vi "Clamp Set.vi"() -> (3 "End":bool)   [LabVIEW 2013]
doc: "This VI is used in 2-ball Autonomous Mode in order to get the second ball from behind the robot."
uses:
  <vilib>/Rock Robotics/WPI/Solenoid/Deprecated/WPI_SolenoidSetBool.vi
panel:
  out "State":T1(ring)
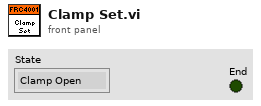
[diagram p1: front panel]
types:
  T1 = enum16{"Clamp Open", "Clamp Down", "Clamp Close", "Clamp Raise"}
  T2 = enum16{"Clamp Open", "Clamp Down", "Clamp Close", "Clamp Raise", "Motor Stop"}
  T3 = typedef "WPI_DigitalInputDevRef.ctl" = cluster{"DevStatus":errorcluster, "DIO Channel":T4, "Digital Module":T5}
  T4 = typedef "FPGA_DIOChannel.ctl" = enum8{"DIO 1", "DIO 2", "DIO 3", "DIO 4", "DIO 5", "DIO 6", "DIO 7", "DIO 8", "DIO 9", "DIO 10", "DIO 11", "DIO 12", "DIO 13", "DIO 14", "Invalid"}
  T5 = typedef "FPGA_TypedefDigitalModule.ctl" = enum16{"Digital Module 1", "Digital Module 2"}
  T6 = typedef "WPI_SolenoidDevRef.ctl" = cluster{"DevStatus":errorcluster, "Solenoid Module":T7, "Forward Solenoid Channel":T8, "Reverse Solenoid Channel":T8}
  T7 = typedef "FPGA_TypedefSolenoidModule.ctl" = enum16{"Solenoid Module 1", "Solenoid Module 2"}
  T8 = typedef "WPI_SolenoidChannel.ctl" = enum8{"Solenoid 1", "Solenoid 2", "Solenoid 3", "Solenoid 4", "Solenoid 5", "Solenoid 6", "Solenoid 7", "Solenoid 8", "Invalid"}
  T9 = typedef "WPI_MotorControlDeviceRef.ctl" = cluster{"DeviceStatus":errorcluster, "Type":enum16{"PWM", "CAN"}, "PWM":cluster{"Digital Module":T5, "PWM Channel":T10, "DeadBand":T11}, "CAN":cluster{"Device Number":u8, "Control Mode":T12, "Semaphore":T13, "Max Vout":dbl}, "Invert":bool, "TransformRef":T14, "InvTransformRef":T14}
  T10 = typedef "FPGA_DIOPWMChannel.ctl" = enum8{"PWM 1", "PWM 2", "PWM 3", "PWM 4", "PWM 5", "PWM 6", "PWM 7", "PWM 8", "PWM 9", "PWM 10", "Invalid"}
  T11 = typedef "WPI_PWMDeadband.ctl" = cluster{"Name":string, "maxPositivePwm":i32, "minPositivePwm":i32, "centerPwm":i32, "maxNegativePwm":i32, "minNegativePwm":i32, "angularRange":u16}
  T12 = typedef "WPI_CANJaguar_ControlMode.ctl" = enum8{"Percent VBus", "Current", "Speed", "Position", "Voltage"}
  T13 = typedef "Semaphore RefNum" = refnum<k1>
  T14 = typedef "WPI_PWMTransform_ConPane.ctl" = refnum<vi>
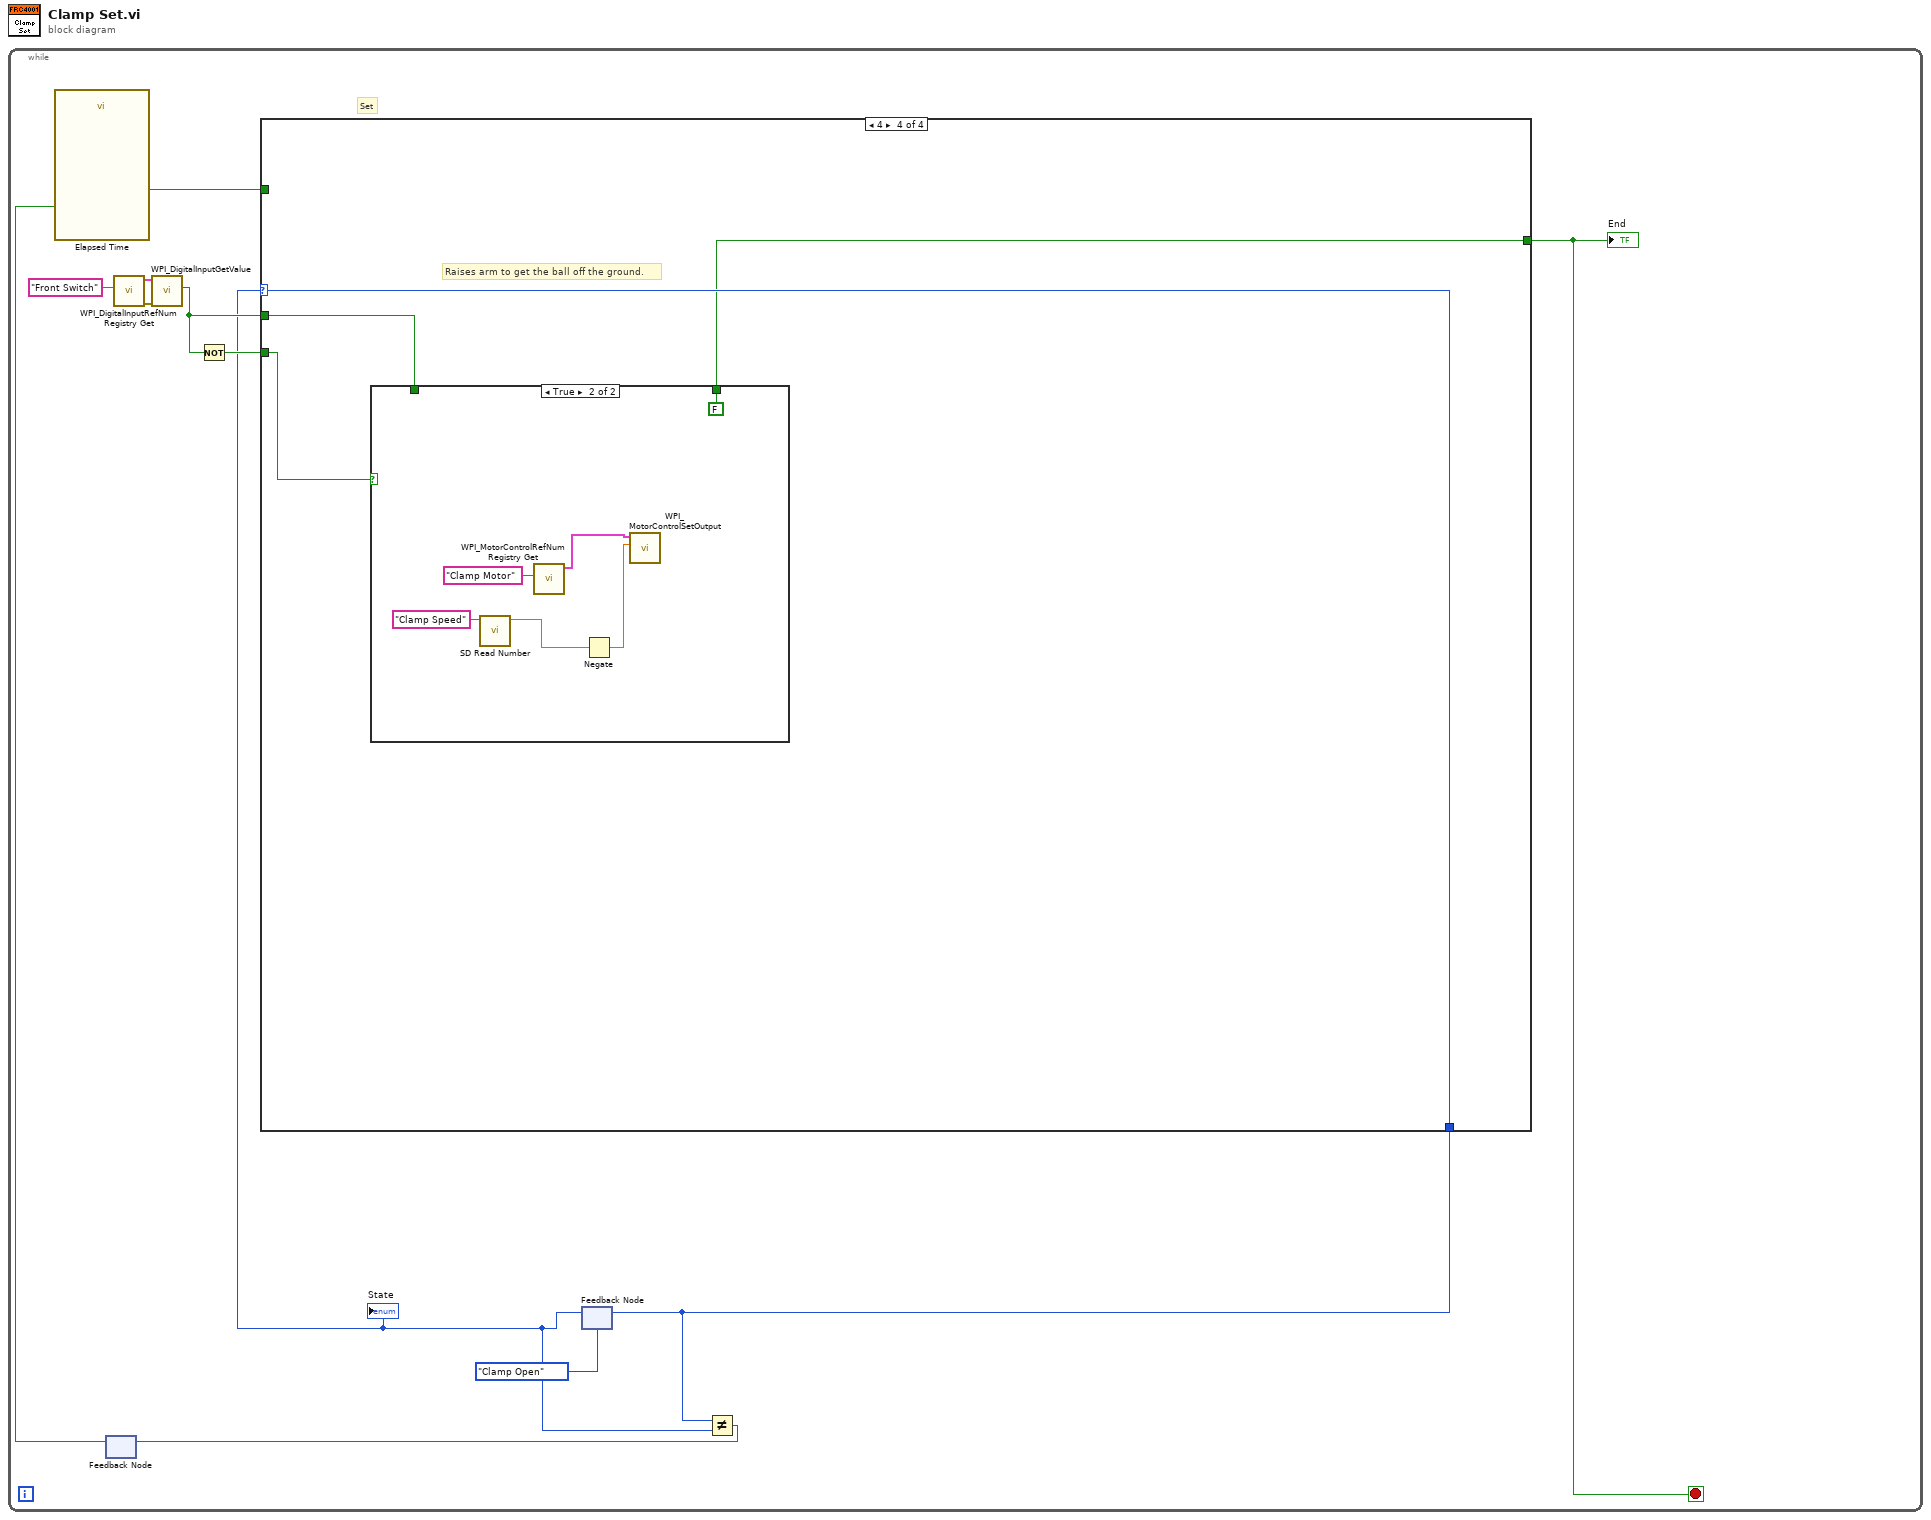
[diagram p0: block diagram]
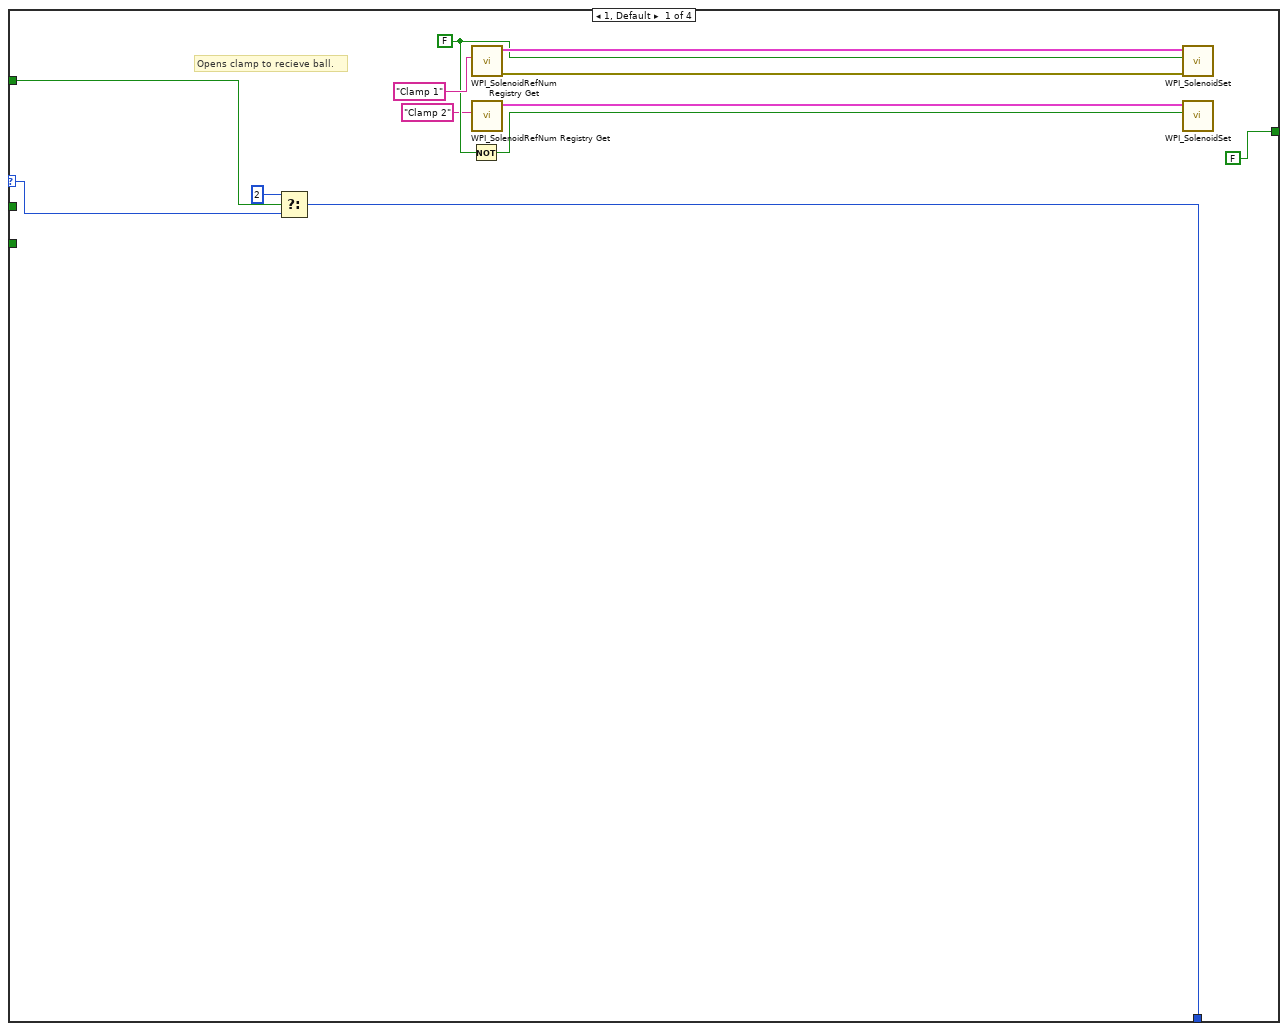
[diagram p2: hidden frame]
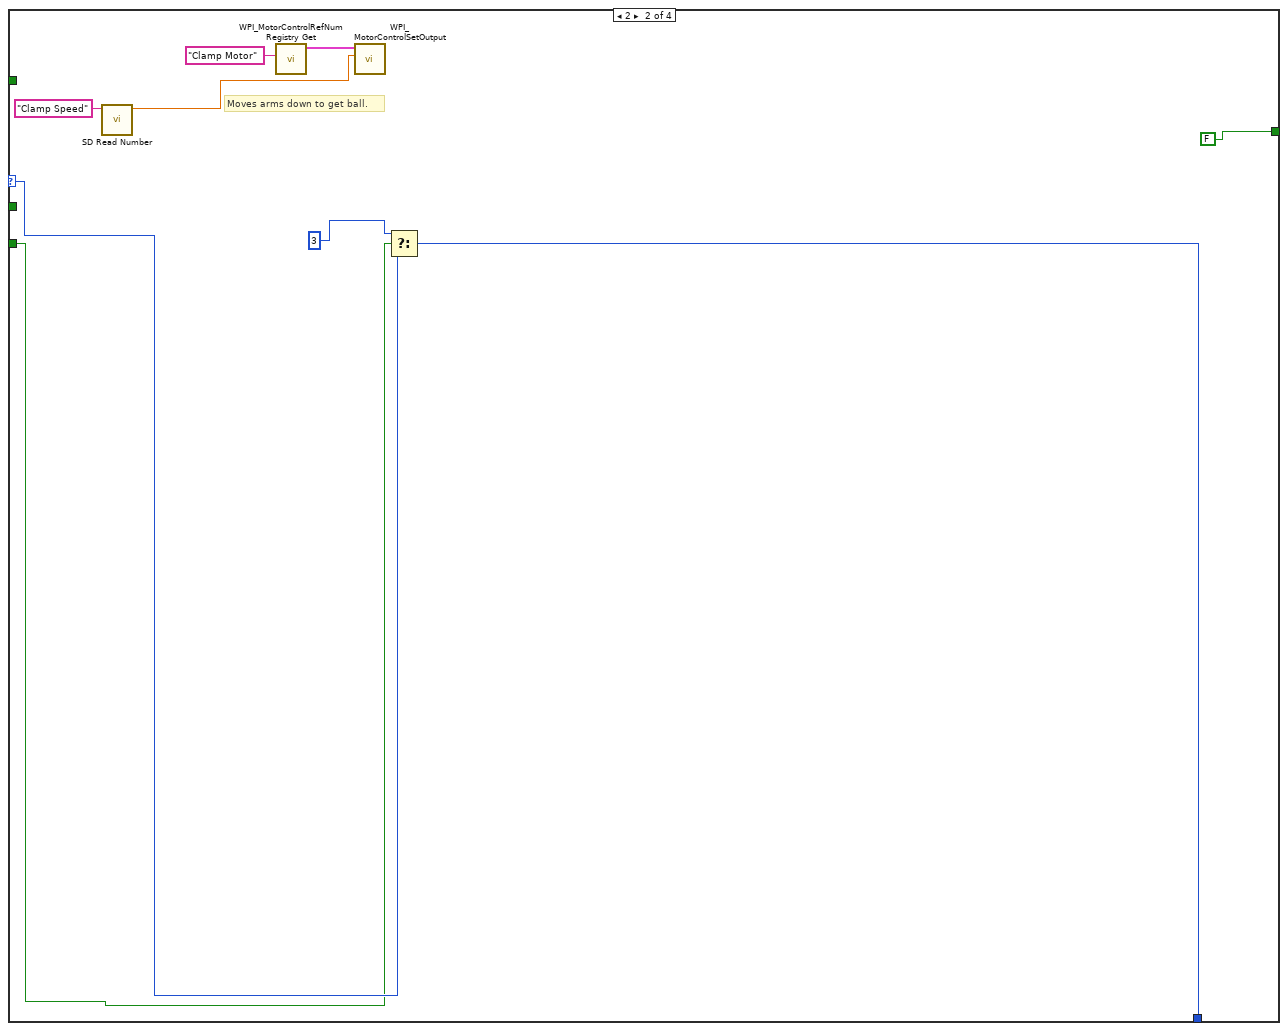
[diagram p3: hidden frame]
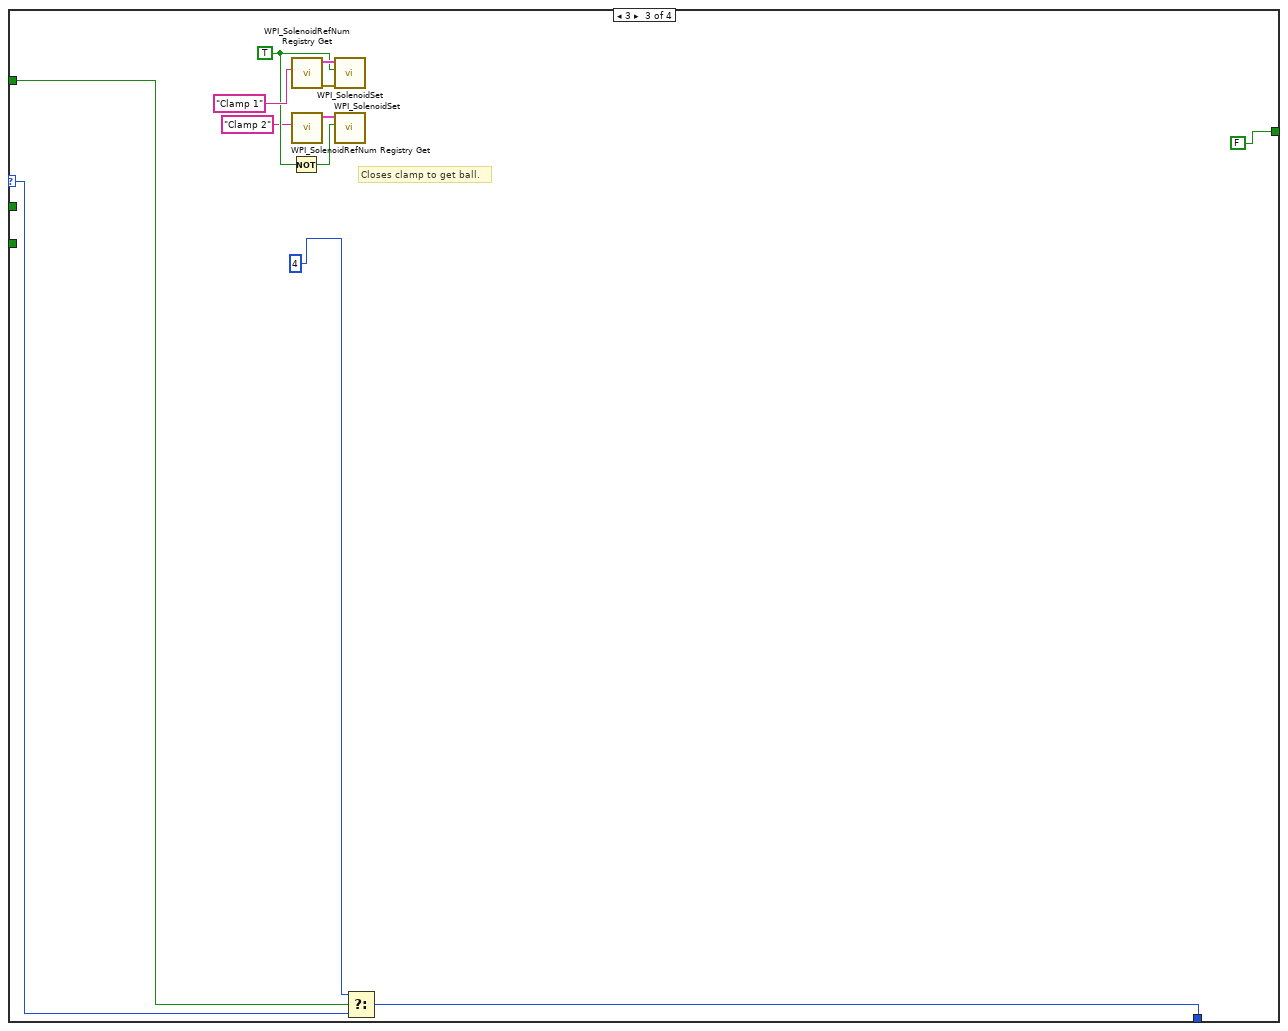
[diagram p4: hidden frame]
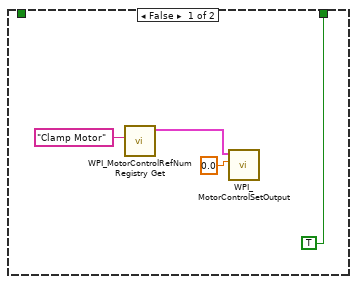
[diagram p5: hidden frame]
diagram:
  n1 = while {
    stop <- w4 stop-if-true
    # "Set"
    n2 = feedback #1() -> (w6:bool)  [unwired: 1 in]
    n3 = call "Elapsed Time"("Reset"=w6) -> ("Time has Elapsed"=w9:bool)  [unwired: 11 in, 7 out]
    n4 = call <vilib>:"WPI_DigitalInputRefNum Registry Get.vi"("refnum name"="Front Switch") -> ("error out"=w11:errorcluster, "DigitalInputDevRef"=w10:T3)  [unwired: 9 in]
    n5 = call <vilib>:"WPI_DigitalInputGetValue.vi"("error in (no error)"=w11, "DigitalInputDevRef"=w10) -> ("Value"=w3:bool)  [unwired: 7 in, 2 out]
    n6 = Not(x=w3) -> (.not. x?=w5:bool)
    n7 = feedback #2(T2."Clamp Open") -> (w1:u16)
    "State" <- w1
    n8 = case shown="4" w1 {
      selector: w1 -> [w23 w32 w44 w49]
      tunnel: [FALSE FALSE FALSE w46] -> w4
      tunnel: [w22 w31 w43 w49] -> w8
      tunnel: w5 -> [_ w28 _ w48]
      tunnel: w9 -> [w14 _ w35 _]
      tunnel: w3 -> [_ _ _ w47]
      frame 1, Default {
        w18 = FALSE
        # "Opens clamp to recieve ball."
        n9 = Select(t=u16 2, s=w14, f=w23) -> (s? t:f=w22:u16)
        n10 = Not(x=w18) -> (.not. x?=w16:bool)
        n11 = call <vilib>:"WPI_SolenoidRefNum Registry Get.vi"("refnum name"="Clamp 1") -> ("error out"=w19:errorcluster, "SolenoidDevRef"=w20:T6)  [unwired: 9 in]
        n12 = call <vilib>:"WPI_SolenoidRefNum Registry Get.vi"("refnum name"="Clamp 2") -> ("SolenoidDevRef"=w17:T6)  [unwired: 9 in, 1 out]
        n13 = call-poly <vilib>:"WPI_SolenoidSet.vi"("error in (no error)"=w19, "Value"=w18, "SolenoidDevRef"=w20) -> ()  [unwired: 7 in, 2 out]
        n14 = call-poly <vilib>:"WPI_SolenoidSet.vi"("Value"=w16, "SolenoidDevRef"=w17) -> ()  [unwired: 8 in, 2 out]
      }
      frame 2 {
        # "Moves arms down to get ball."
        n15 = call <vilib>:"SD Read Number.vi"("Name"="Clamp Speed") -> ("Numeric"=w25:dbl)  [unwired: 8 in, 2 out]
        n16 = call <vilib>:"WPI_MotorControlRefNum Registry Get.vi"("refnum name"="Clamp Motor") -> ("MotorControlDevRef"=w29:T9)  [unwired: 9 in, 1 out]
        n17 = call <vilib>:"WPI_MotorControlSetOutput.vi"("Output"=w25, "MotorControlDevRef"=w29) -> ()  [unwired: 7 in, 3 out]
        n18 = Select(t=u16 3, s=w28, f=w32) -> (s? t:f=w31:u16)
      }
      frame 3 {
        w39 = TRUE
        # "Closes clamp to get ball."
        n19 = Not(x=w39) -> (.not. x?=w37:bool)
        n20 = call <vilib>:"WPI_SolenoidRefNum Registry Get.vi"("refnum name"="Clamp 1") -> ("error out"=w40:errorcluster, "SolenoidDevRef"=w41:T6)  [unwired: 9 in]
        n21 = call <vilib>:"WPI_SolenoidRefNum Registry Get.vi"("refnum name"="Clamp 2") -> ("SolenoidDevRef"=w38:T6)  [unwired: 9 in, 1 out]
        n22 = call-poly <vilib>:"WPI_SolenoidSet.vi"("error in (no error)"=w40, "Value"=w39, "SolenoidDevRef"=w41) -> ()  [unwired: 7 in, 2 out]
        n23 = call-poly <vilib>:"WPI_SolenoidSet.vi"("Value"=w37, "SolenoidDevRef"=w38) -> ()  [unwired: 8 in, 2 out]
        n24 = Select(t=u16 4, s=w35, f=w44) -> (s? t:f=w43:u16)
      }
      frame 4 {
        # "Raises arm to get the ball off the ground."
        n25 = case shown="True" w48 {
          tunnel: w47 -> [_ _]
          tunnel: [TRUE FALSE] -> w46
          frame False {
            n26 = call <vilib>:"WPI_MotorControlRefNum Registry Get.vi"("refnum name"="Clamp Motor") -> ("MotorControlDevRef"=w51:T9)  [unwired: 9 in, 1 out]
            n27 = call <vilib>:"WPI_MotorControlSetOutput.vi"("Output"=0.0, "MotorControlDevRef"=w51) -> ()  [unwired: 7 in, 3 out]
          }
          frame True {
            n28 = call <vilib>:"SD Read Number.vi"("Name"="Clamp Speed") -> ("Numeric"=w54:dbl)  [unwired: 8 in, 2 out]
            n29 = call <vilib>:"WPI_MotorControlRefNum Registry Get.vi"("refnum name"="Clamp Motor") -> ("MotorControlDevRef"=w58:T9)  [unwired: 9 in, 1 out]
            n30 = Negate(x=w54) -> (-x=w56:dbl)
            n31 = call <vilib>:"WPI_MotorControlSetOutput.vi"("Output"=w56, "MotorControlDevRef"=w58) -> ()  [unwired: 7 in, 3 out]
          }
        }
      }
    }
    "End" <- w4
    n32 = feedback-in #2(w8) -> ()
    n33 = Not Equal?(x=w8, y=w1) -> (x != y?=w7:bool)
    n34 = feedback-in #1(w7) -> ()
  }
